vi "GA Set Pos.vi"(8 "error in (no error)":errorcluster caption="错误输入（无错误）", 10 "pos":i32, 11 "nAxisNum":i16) -> (0 "error out":errorcluster caption="错误输出", 3 "function return":i32)   [LabVIEW 2024, in "GAS.lvlib"]
doc: "extern \"C\" __declspec(dllimport) int GA_SetPos(short nAxisNum,long pos);"
uses:
  GAS.lvlib
  GAS.dll
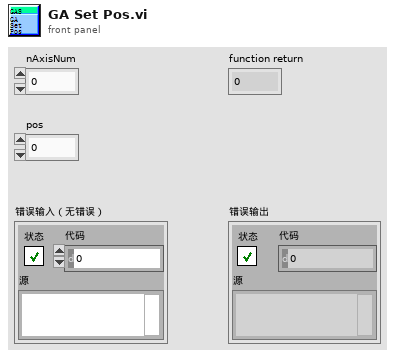
[diagram p1: front panel]
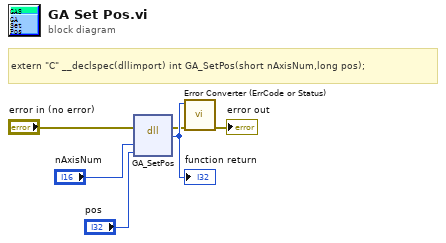
[diagram p0: block diagram]
diagram:
  # "extern \"C\" __declspec(dllimport) int GA_SetPos(short nAxisNum,long pos);"
  n1 = dll-call lib="PTH2?abs D实验室软件（勿删）集成测试系统GAS.*" fn="GA_SetPos"(error in="error in (no error)", "nAxisNum"="nAxisNum", "pos"="pos") -> (error out=w2:errorcluster, w6:i32)  [unwired: 4 in, 1 out]
  "function return" <- w6
  n2 = call "Error Converter (ErrCode or Status).vi"("error in (no error)"=w2, "error code"=w6) -> ("error out"=→"error out":errorcluster)  [unwired: 9 in]
